vi "StoreViRef(SubVI).vi"(9 "Previous 2":refnum<vi>, 10 "Next 2":refnum<vi>, 11 "vi reference":refnum<vi>) -> (3 "Array":refnum<vi>[](array[refnum]))   [LabVIEW 2013]
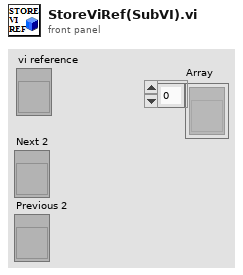
[diagram p1: front panel]
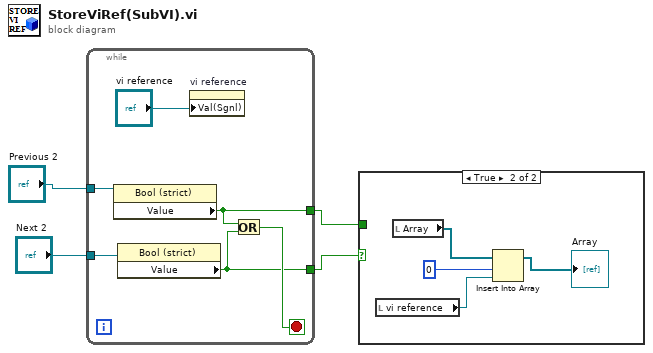
[diagram p0: block diagram]
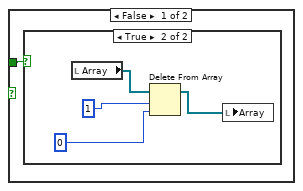
[diagram p2: hidden frame]
diagram:
  n1 = while {
    tunnel: "Next 2" -> [w8]
    tunnel: "Previous 2" -> [w9]
    tunnel: [w6] -> w1
    tunnel: [w5] -> w2
    stop <- w7 stop-if-true
    n2 = property class="Bool (strict)"(reference=w9) -> ("Value"=w6:bool)  [unwired: 1 in, 2 out]
    n3 = property class="Bool (strict)"(reference=w8) -> ("Value"=w5:bool)  [unwired: 1 in, 2 out]
    n4 = property on="vi reference" class="VIRef (strict)"("Val(Sgnl)"="vi reference") -> ()  [unwired: 2 in, 2 out]
    n5 = Or(x=w6, y=w5) -> (x .or. y?=w7:bool)
  }
  n6 = case shown="True" w2 {
    tunnel: w1 -> [w11 _]
    frame False {
      n7 = case shown="True" w11 {
        frame False {
        }
        frame True {
          n8 = local read "Array"() -> (w14:refnum<vi>[])
          n9 = Delete From Array(array=w14, length=1, index=0) -> (array with subset deleted=w15:refnum<vi>[])  [unwired: 1 out]
          n10 = local write "Array"(w15) -> ()
        }
      }
    }
    frame True {
      n11 = local read "vi reference"() -> (w17:refnum<vi>)
      n12 = local read "Array"() -> (w18:refnum<vi>[])
      n13 = Insert Into Array(array=w18, index=0, new element=w17) -> (→"Array":refnum<vi>[])
    }
  }
